vi "DO.vi"() -> ()   [LabVIEW 2010]
panel:
  in  "数值out1 2":dbl min=0.0 max=3.0
  in  "索引 2":i32
  in  "索引":i32
  out "数值in2":dbl min=0.0 max=3.0
  out "数值in1":dbl min=0.0 max=3.0
  out "数值":dbl
  in  "字符串":string
  in  "置0":bool
  in  "置1":bool
  out "停止":bool
  in  "确定按钮":bool
  in  "数值out1":dbl min=0.0 max=3.0
  out "DI8~DI15":bool[](array[boolean])
  out "DI0~DI7":bool[](array[boolean])
  in  "停止":bool
  in  "数组 2":bool[](array[boolean])
  in  "数组":bool[](array[boolean])
  # "DO8---43"
  # "DO0---47"
  # "DO1---13"
  # "DO7"
  # "DO15"
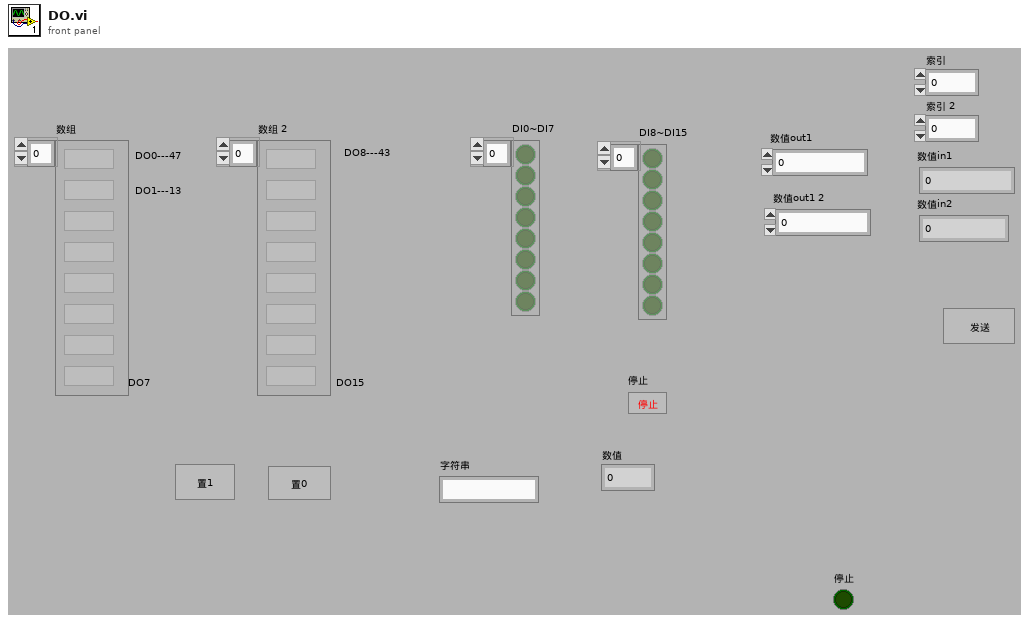
[diagram p1: front panel]
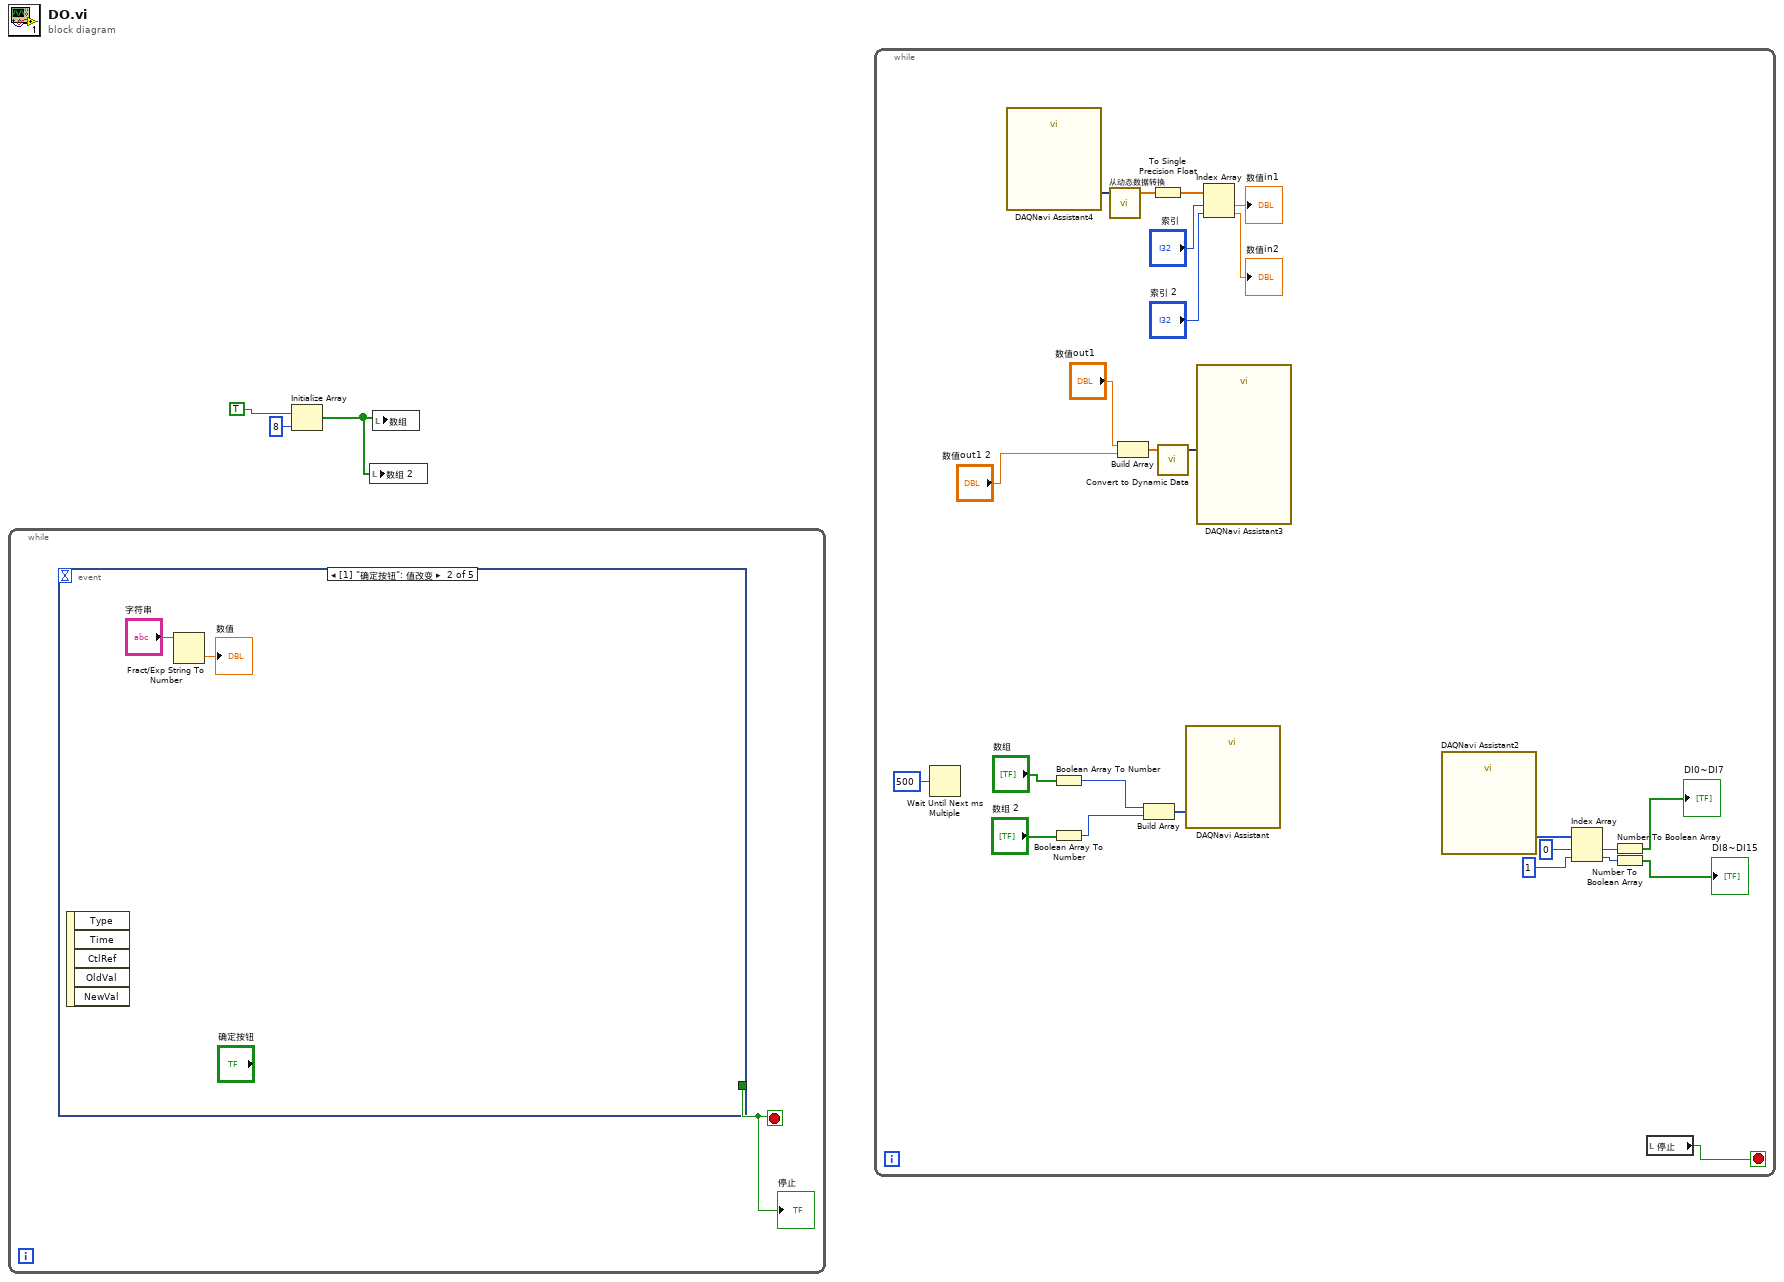
[diagram p0: block diagram]
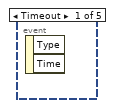
[diagram p2: hidden frame]
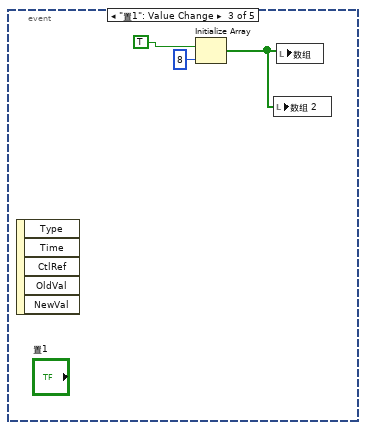
[diagram p3: hidden frame]
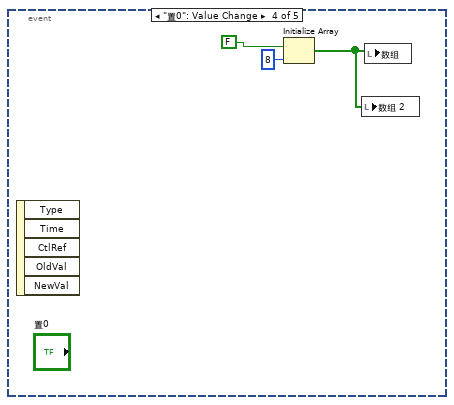
[diagram p4: hidden frame]
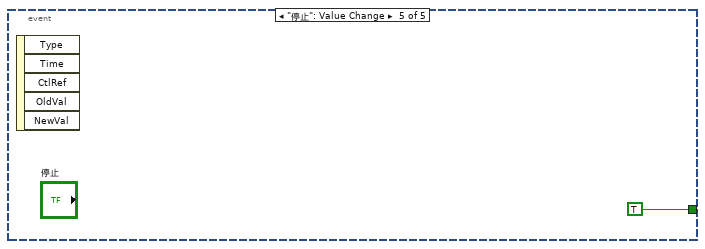
[diagram p5: hidden frame]
diagram:
  n1 = while {
    stop <- w4 stop-if-true
    n2 = event shown="[1] \"确定按钮\": 值改变" {
      selector: _ -> [_ _ _ _ _]
      dyn-events: _ -> [_ _ _ _ _]
      timeout: _ -> [_ _ _ _ _]
      tunnel: [_ _ _ _ TRUE] -> w4
      event Timeout {
        n3 = event-data() -> ()  [unwired: 1 in, 2 out]
      }
      event "确定按钮": Value Change {
        n4 = event-data() -> ()  [unwired: 1 in, 5 out]
        n5 = Fract/Exp String To Number(string="字符串") -> (number=→"数值":dbl)  [unwired: 3 in, 1 out]
      }
      event "置1": Value Change {
        n6 = event-data() -> ()  [unwired: 1 in, 5 out]
        n7 = Initialize Array(TRUE, 8 ("维数大小")) -> (w7:bool[])
        n8 = local write "数组 2"(w7) -> ()
        n9 = local write "数组"(w7) -> ()
      }
      event "置0": Value Change {
        n10 = event-data() -> ()  [unwired: 1 in, 5 out]
        n11 = Initialize Array(FALSE, 8 ("维数大小")) -> (w10:bool[])
        n12 = local write "数组 2"(w10) -> ()
        n13 = local write "数组"(w10) -> ()
      }
      event "停止": Value Change {
        n14 = event-data() -> ()  [unwired: 1 in, 5 out]
      }
    }
    "停止" <- w4
  }
  n15 = Initialize Array(TRUE, 8 ("维数大小")) -> (w3:bool[])
  n16 = local write "数组 2"(w3) -> ()
  n17 = local write "数组"(w3) -> ()
  n18 = while {
    stop <- w26 stop-if-true
    n19 = Wait Until Next ms Multiple(millisecond multiple=u32 500 ("毫秒倍数")) -> ()  [unwired: 1 out]
    n20 = call "DAQNavi Assistant4"() -> ("data out(DDT)"=w19:dynamicdata)  [unwired: 2 in, 17 out]
    n21 = Boolean Array To Number ("布尔数组至数值转换")(Boolean array="数组") -> (number=w27:u8)
    n22 = Boolean Array To Number ("布尔数组至数值转换")(Boolean array="数组 2") -> (number=w28:u8)
    n23 = call "从动态数据转换"("Dynamic Data Type"=w19) -> ("Array"=w20:dbl[])  [unwired: 3 in]
    n24 = Build Array("数值out1", "数值out1 2") -> (w17:dbl[])
    n25 = Build Array(w27, w28) -> (w30:u8[])
    n26 = To Single Precision Float(number=w20) -> (single precision float=w21:sgl[])
    n27 = call "Convert to Dynamic Data"("Array"=w17) -> ("Dynamic Data Type"=w16:dynamicdata)  [unwired: 3 out]
    n28 = call "DAQNavi Assistant"("dataIn(U8Array)"=w30) -> ()  [unwired: 2 in, 17 out]
    n29 = call "DAQNavi Assistant3"("data in(DDT)"=w16) -> ()  [unwired: 2 in, 17 out]
    n30 = Index Array(array=w21, index #1="索引", index #2="索引 2") -> (element #1=→"数值in1":sgl, element #2=→"数值in2":sgl)
    n31 = call "DAQNavi Assistant2"() -> ("dataOut(U8Array)"=w37:u8[])  [unwired: 2 in, 17 out]
    n32 = Index Array(array=w37, index #1=0 ("索引"), index #2=1 ("索引")) -> (element #1=w34:u8, element #2=w33:u8)
    n33 = Number To Boolean Array(number=w34) -> (Boolean array=→"DI0~DI7":bool[])
    n34 = Number To Boolean Array(number=w33) -> (Boolean array=→"DI8~DI15":bool[])
    n35 = local read "停止"() -> (w26:bool)
  }
